vi "DMSV.main.vi"() -> ()   [LabVIEW 2014, in "DMSViewer.lvlib"]
doc: "Displays node and processs information as well as status of CS systems.\n\nHistory: 16-FEB-2006, Dietrich Beck\n\nCopyright (C)\nGesellschaft für Schwerionenforschung, GSI\nPlanckstr. 1\n64291 Darmstadt\nGermany\n\nContact: D.Beck@gsi.de \n\nThis program is free software; you can redistribute it and/or modify it under the terms of the \nGNU General Public License as published by the Free Software Foundation; either version 2 of the license, or (at your option) any later version.\n\nThis program is distributed in the hope that it will be useful, but WITHOUT ANY WARRANTY; without even the implied warranty of MERCHANTABILITY or FITNESS FOR A PARTICULAR PURPOSE. See the GNU General License for more details (http://www.gnu.org).\n\nGesellschaft für Schwerionenforschung, GSI\nPlanckstr. 1, 64291 Darmstadt, Germany\nFor all questions and ideas contact D. Beck.\nLast update: 16-DEC-2005"
uses:
  DMSViewer.lvlib
  CSlibraries-extern/DimLVEvent/LVDimInterface/LVDimInterface.dim service type.ctl
  CSlibraries/UtilityLib/UtilityLib.valueStatus.ctl
  CSlibraries-extern/DimLVEvent/LVDimInterface/LVDimInterface.dic_info_service_notifier.vi
  CSlibraries-extern/DimLVEvent/LVDimInterface/LVDimInterface.lvlib
  CSlibraries/UtilityLib/UtilityLib.lvlib
panel:
  out "nameAndVersion":string
  out "domainMessage":string
  in  "ShowCSSystems":bool
  out "CSSystems":i32(listbox)=-1
  out "noLink":bool
  in  "DomainName":string="KSTest"
  in  "setDomain":bool
  in  "Nodes":i32(listbox)
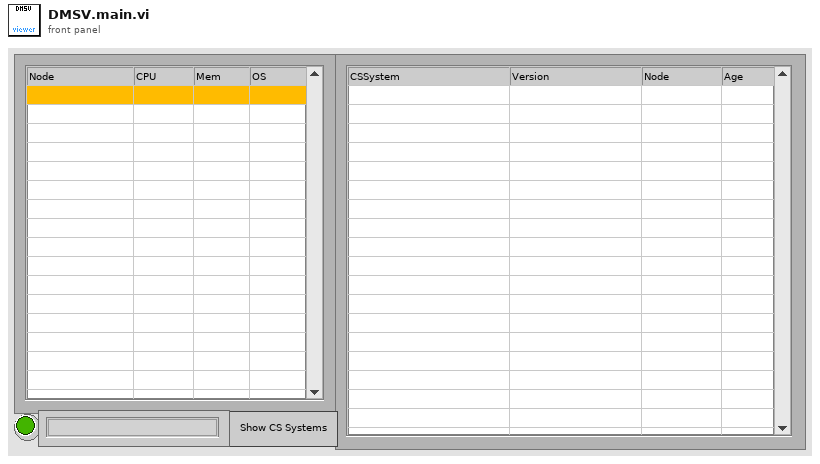
[diagram p1: front panel]
types:
  T1 = typedef "UtilityLib.lvlib/UtilityLib.valueStatus.ctl" = enum16{"no info available", "stand by/off", "on", "warning", "alarm/malfunction", "not implemented", "user action required", "important information", "system default", "control default", "indicator default", "button default"}
  T2 = enum32{"invalid app kind", "Development System", "Run Time System", "Student Edition", "Embedded LabVIEW", "Evaluation", "Custom"}
  T3 = typedef "LVDimInterface.lvlib/LVDimInterface.dim service type.ctl" = u16
  T4 = typedef "LVRectTypeDef.ctl" = cluster{"Left":i16, "Top":i16, "Right":i16, "Bottom":i16}
  T5 = typedef "LVPointTypeDef.ctl" = cluster{"Horizontal":i16, "Vertical":i16}
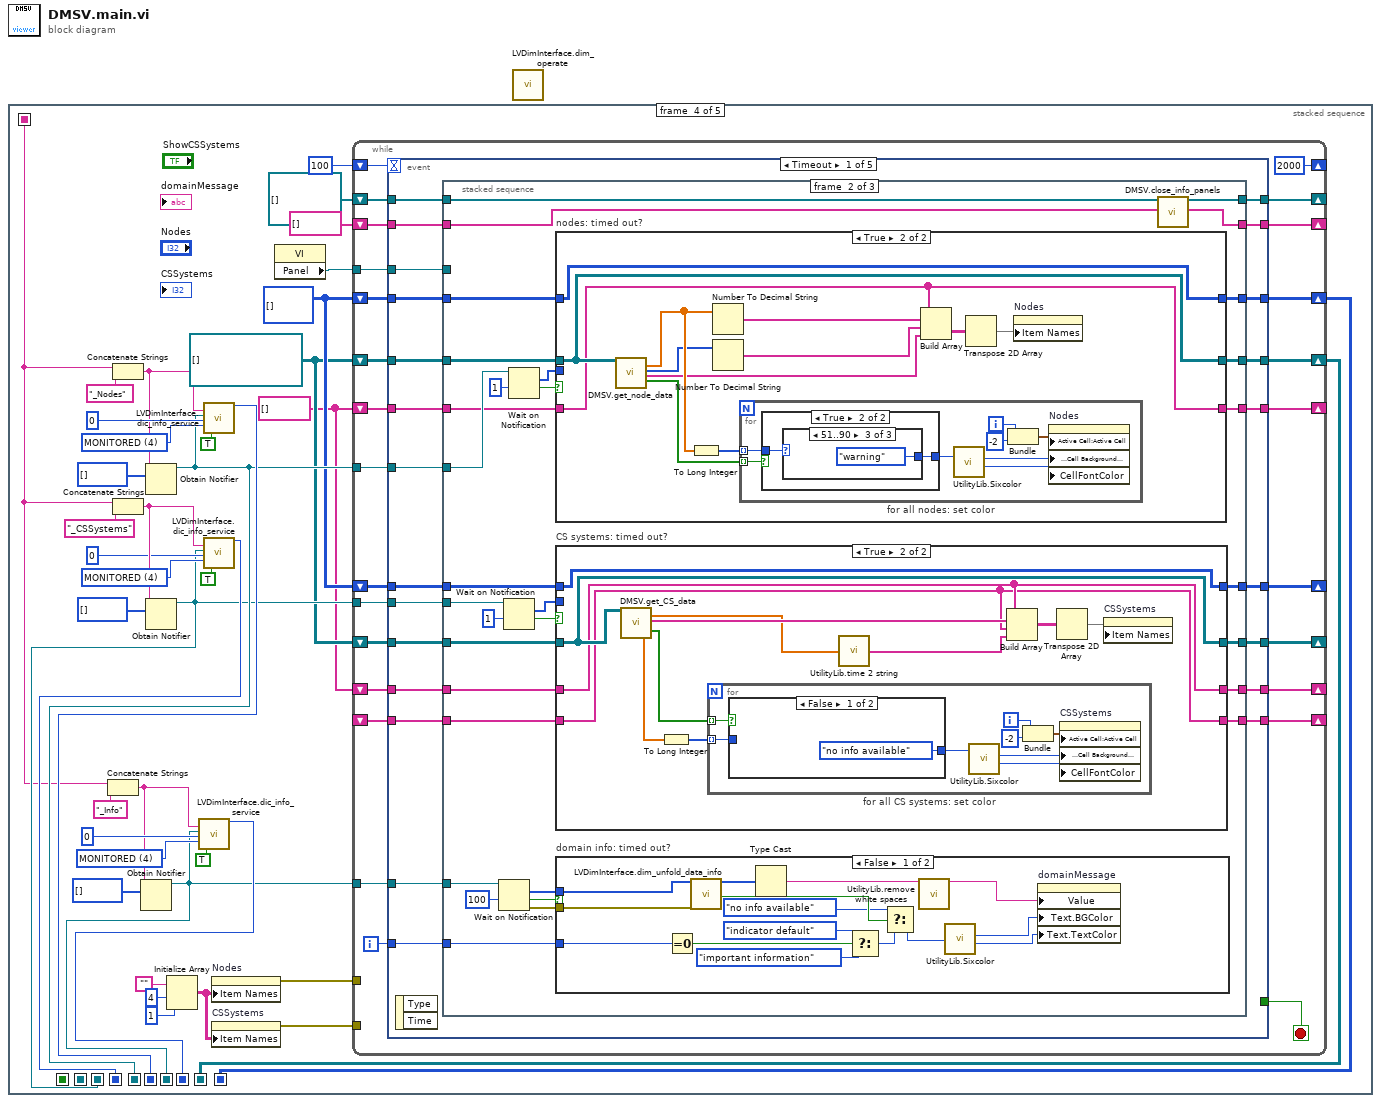
[diagram p0: block diagram]
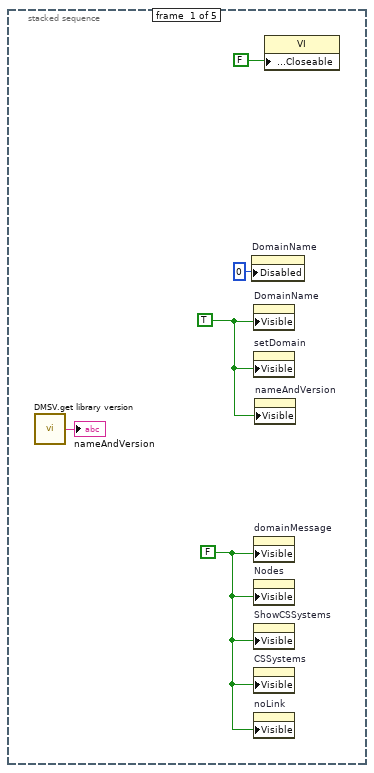
[diagram p2: hidden frame]
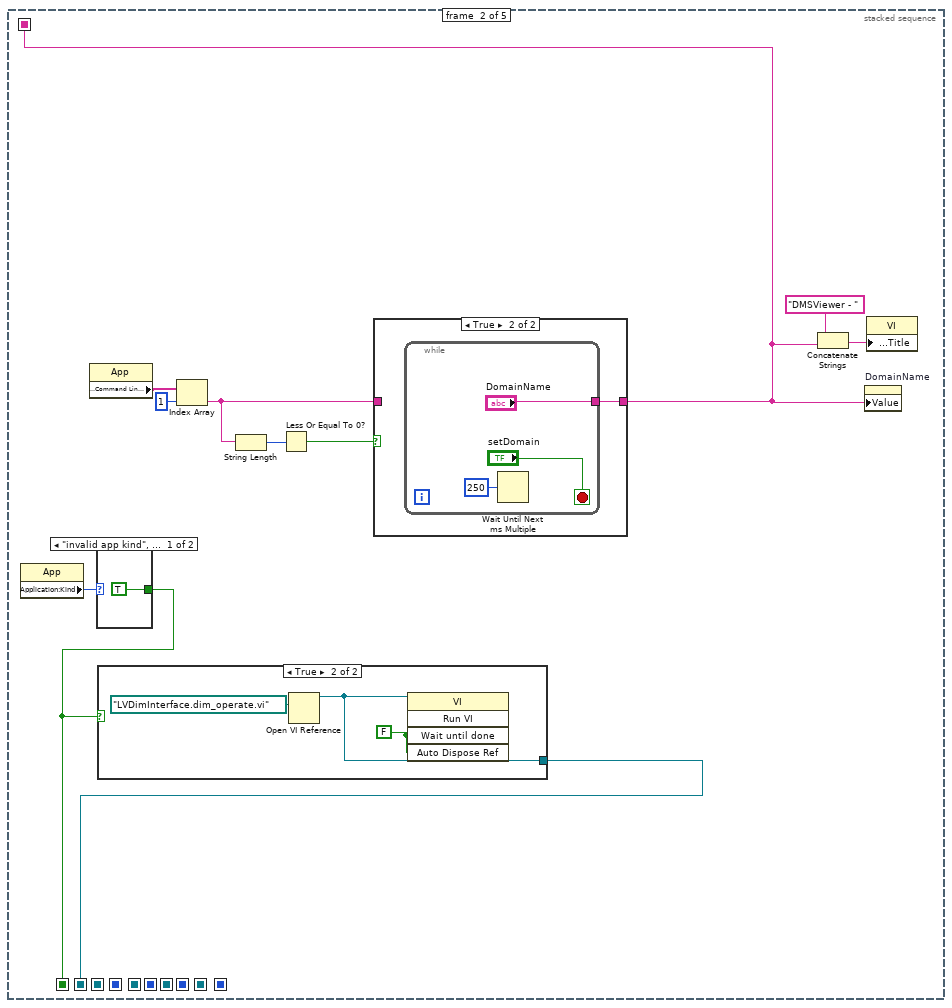
[diagram p3: hidden frame]
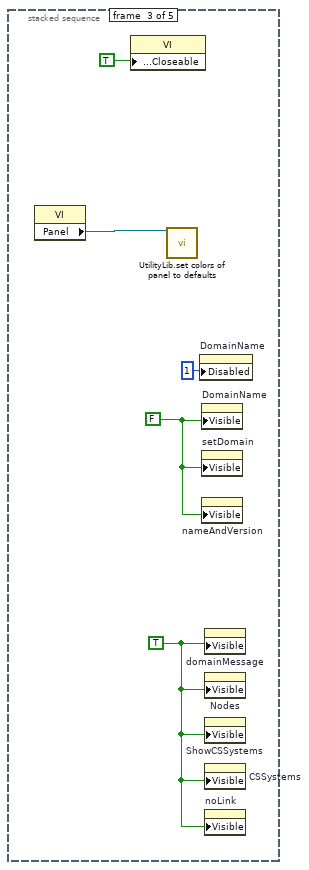
[diagram p7: hidden frame]
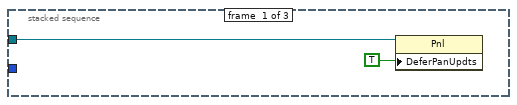
[diagram p8: hidden frame]
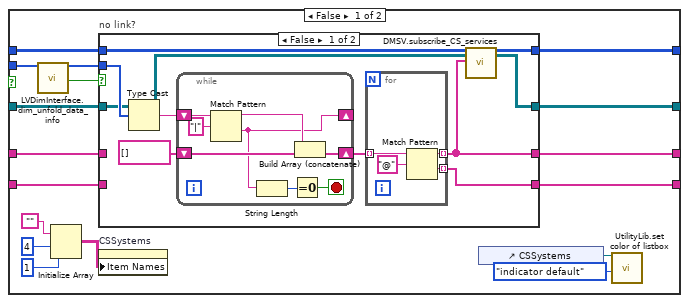
[diagram p10: hidden frame]
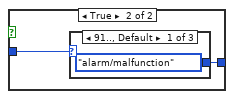
[diagram p12: hidden frame]
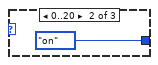
[diagram p13: hidden frame]
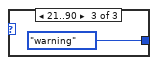
[diagram p14: hidden frame]
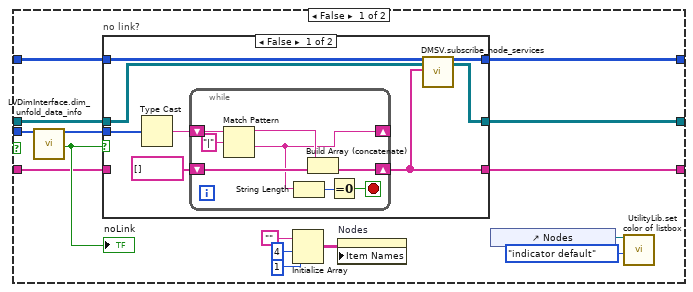
[diagram p15: hidden frame]
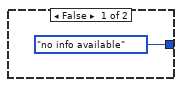
[diagram p17: hidden frame]
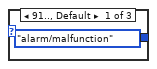
[diagram p18: hidden frame]
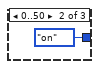
[diagram p19: hidden frame]
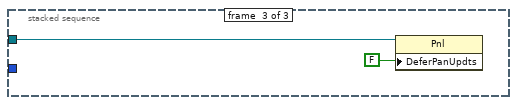
[diagram p20: hidden frame]
diagram:
  n1 = stacked-sequence {
    seq-local: [_ w7 _ _ _] -> [_ _ _ w33 _]
    seq-local: [_ w9 _ _ _] -> [_ _ _ _ w398]
    seq-local: [_ w11 _ _ _] -> [_ _ _ _ w397]
    seq-local: [_ _ _ w54 _] -> [_ _ _ _ w394]
    seq-local: [_ _ _ w59 _] -> [_ _ _ _ w396]
    seq-local: [_ _ _ w56 _] -> [_ _ _ _ w392]
    seq-local: [_ _ _ w55 _] -> [_ _ _ _ w393]
    seq-local: [_ _ _ w47 _] -> [_ _ _ _ w389]
    seq-local: [_ _ _ w46 _] -> [_ _ _ _ w390]
    seq-local: [_ _ _ w31 _] -> [_ _ _ _ w387]
    seq-local: [_ _ _ w32 _] -> [_ _ _ _ w386]
    frame #0 {
      w4 = FALSE ("Visible")
      w1 = TRUE ("Visible")
      n2 = call "DMSV.get library version.vi"() -> ("nameAndVersion"=→"nameAndVersion":string)  [unwired: 1 in]
      n3 = property on="DomainName" class="Str"("Disabled"=u8 0) -> ()  [unwired: 2 in, 2 out]
      n4 = property on="DomainName" class="Str"("Visible"=w1) -> ()  [unwired: 2 in, 2 out]
      n5 = property on="setDomain" class="Bool"("Visible"=w1) -> ()  [unwired: 2 in, 2 out]
      n6 = property on="domainMessage" class="Str"("Visible"=w4) -> ()  [unwired: 2 in, 2 out]
      n7 = property on="Nodes" class="MCListbox (strict)"("Visible"=w4) -> ()  [unwired: 2 in, 2 out]
      n8 = property on="ShowCSSystems" class="Bool (strict)"("Visible"=w4) -> ()  [unwired: 2 in, 2 out]
      n9 = property on="CSSystems" class="MCListbox (strict)"("Visible"=w4) -> ()  [unwired: 2 in, 2 out]
      n10 = property on="noLink" class="Bool (strict)"("Visible"=w4) -> ()  [unwired: 2 in, 2 out]
      n11 = property on="nameAndVersion" class="Str"("Visible"=w1) -> ()  [unwired: 2 in, 2 out]
      n12 = property class="VI"("Front Panel.Closeable"=FALSE ("Front Panel Window:Closeable")) -> ()  [unwired: 2 in, 2 out]
    }
    frame #1 {
      n13 = property on="Property Node" class="App"() -> ("Application:Kind"=w10:T2)  [unwired: 2 in, 2 out]
      n14 = property on="Property Node" class="App"() -> ("Application:Command Line Arguments"=w16:string[])  [unwired: 2 in, 2 out]
      n15 = case shown="\"invalid app kind\", Default" w10 {
        tunnel: [TRUE _] -> w9
        frame "invalid app kind", Default {
        }
        frame "Development System" {
        }
      }
      n16 = case shown="True" w9 {
        tunnel: [_ w18] -> w11
        frame False {
        }
        frame True {
          w19 = FALSE ("Wait until done")
          n17 = Open VI Reference(vi path=path "LVDimInterface.dim_operate.vi") -> (vi reference=w18:refnum<vi>)  [unwired: 5 in, 1 out]
          n18 = invoke on="Invoke Node" class="VI" method="Run VI"(reference=w18, "Wait until done"=w19, "Auto Dispose Ref"=w19) -> ()  [unwired: 2 in, 5 out]
        }
      }
      n19 = Index Array(array=w16, index=1) -> (element=w12:string)
      n20 = String Length(string=w12) -> (length=w14:i32)
      n21 = Less Or Equal To 0?(x=w14) -> (x <= 0?=w13:bool)
      n22 = case shown="True" w13 {
        tunnel: [w21 w22] -> w7
        tunnel: w12 -> [w21 _]
        frame False {
        }
        frame True {
          n23 = while {
            tunnel: ["DomainName"] -> w22
            stop <- "setDomain" stop-if-true
            n24 = Wait Until Next ms Multiple(millisecond multiple=u32 250) -> ()  [unwired: 1 out]
          }
        }
      }
      n25 = Concatenate Strings("DMSViewer - " ("string"), w7) -> (w8:string)
      n26 = property on="DomainName" class="Str"("Value"=w7) -> ()  [unwired: 2 in, 2 out]
      n27 = property on="Property Node" class="VI"("Front Panel Window:Title"=w8) -> ()  [unwired: 2 in, 2 out]
    }
    frame #2 {
      w29 = TRUE ("Visible")
      w26 = FALSE ("Visible")
      n28 = property on="Property Node" class="VI"() -> ("Panel"=w28:refnum<vi>)  [unwired: 2 in, 2 out]
      n29 = property class="VI"("Front Panel.Closeable"=TRUE ("Front Panel Window:Closeable")) -> ()  [unwired: 2 in, 2 out]
      n30 = call "UtilityLib.set colors of panel to defaults.vi"("Front Panel"=w28) -> ()  [unwired: 18 in, 1 out]
      n31 = property on="DomainName" class="Str"("Disabled"=u8 1) -> ()  [unwired: 2 in, 2 out]
      n32 = property on="DomainName" class="Str"("Visible"=w26) -> ()  [unwired: 2 in, 2 out]
      n33 = property on="setDomain" class="Bool"("Visible"=w26) -> ()  [unwired: 2 in, 2 out]
      n34 = property on="nameAndVersion" class="Str"("Visible"=w26) -> ()  [unwired: 2 in, 2 out]
      n35 = property on="domainMessage" class="Str"("Visible"=w29) -> ()  [unwired: 2 in, 2 out]
      n36 = property on="Nodes" class="MCListbox (strict)"("Visible"=w29) -> ()  [unwired: 2 in, 2 out]
      n37 = property on="ShowCSSystems" class="Bool (strict)"("Visible"=w29) -> ()  [unwired: 2 in, 2 out]
      n38 = property on="CSSystems" class="MCListbox (strict)"("Visible"=w29) -> ()  [unwired: 2 in, 2 out]
      n39 = property on="noLink" class="Bool (strict)"("Visible"=w29) -> ()  [unwired: 2 in, 2 out]
    }
    frame #3 {
      w36 = T3 4 items=["ONCE_ONLY"=1, "TIMED"=2, "MONITORED"=4] ("serviceType")
      w43 = string[] []
      w51 = T3 4 items=["ONCE_ONLY"=1, "TIMED"=2, "MONITORED"=4] ("serviceType")
      w44 = refnum<notifier>[][] [] ("nodeNotifiers (out)")
      w45 = i32[][] [] ("nodeServices (out)")
      w60 = T3 4 items=["ONCE_ONLY"=1, "TIMED"=2, "MONITORED"=4] ("serviceType")
      n40 = Concatenate Strings(w33, "_Info" ("string")) -> (w34:string)
      n41 = Concatenate Strings(w33, "_Nodes" ("string")) -> (w57:string)
      n42 = Concatenate Strings(w33, "_CSSystems" ("string")) -> (w53:string)
      n43 = Obtain Notifier(name (unnamed)=w34, notification data type=i8[] []) -> (notifier out=w31:refnum<notifier>)  [unwired: 2 in, 2 out]
      n44 = Obtain Notifier(name (unnamed)=w57, notification data type=i8[] []) -> (notifier out=w54:refnum<notifier>)  [unwired: 2 in, 2 out]
      n45 = Obtain Notifier(name (unnamed)=w53, notification data type=i8[] []) -> (notifier out=w46:refnum<notifier>)  [unwired: 2 in, 2 out]
      n46 = Initialize Array("" ("Empty String Constant"), 4 ("dimension size"), 1 ("dimension size")) -> (w42:string[][])
      n47 = call-poly "LVDimInterface.dic_info_service.vi"("serviceName"=w34, "notifierRef"=w31, "timeout [s]"=0, "serviceType"=w36, "stamped"=TRUE) -> ("callBackID"=w32:i32)  [unwired: 13 in, 1 out]
      n48 = call-poly "LVDimInterface.dic_info_service.vi"("serviceName"=w57, "notifierRef"=w54, "timeout [s]"=0, "serviceType"=w60, "stamped"=TRUE) -> ("callBackID"=w59:i32)  [unwired: 13 in, 1 out]
      n49 = call-poly "LVDimInterface.dic_info_service.vi"("serviceName"=w53, "notifierRef"=w46, "timeout [s]"=0, "serviceType"=w51, "stamped"=TRUE) -> ("callBackID"=w47:i32)  [unwired: 13 in, 1 out]
      n50 = property on="Nodes" class="MCListbox (strict)"("Item Names"=w42) -> (error out=w69:errorcluster)  [unwired: 2 in, 1 out]
      n51 = property on="CSSystems" class="MCListbox (strict)"("Item Names"=w42) -> (error out=w41:errorcluster)  [unwired: 2 in, 1 out]
      n52 = property on="Property Node" class="VI"() -> ("Panel"=w40:refnum<vi>)  [unwired: 2 in, 2 out]
      n53 = while {
        shift-right: [w94] -> _
        shift-left: refnum<vi>[] [] -> [w95]
        tunnel: w69 -> [_]
        shift-right: [2000] -> _
        shift-left: 100 -> [w92]
        shift-right: [w90] -> _
        shift-left: string[] [] -> [w91]
        tunnel: w54 -> [w89]
        shift-right: [w88] -> w55
        shift-left: w45 -> [w86]
        shift-right: [w87] -> w56
        shift-left: w44 -> [w85]
        shift-right: [w84] -> _
        shift-left: w43 -> [w83]
        tunnel: w46 -> [w82]
        shift-right: [w80] -> _
        shift-left: w45 -> [w77]
        shift-right: [w79] -> _
        shift-left: w44 -> [w78]
        shift-right: [w81] -> _
        shift-left: w43 -> [w71]
        tunnel: w41 -> [_]
        shift-right: [w76] -> _
        shift-left: _ -> [w75]
        tunnel: w40 -> [w74]
        tunnel: w31 -> [w73]
        i -> [w72]
        stop <- w96 stop-if-true
        n54 = event shown="[0] Timeout" {
          selector: _ -> [_ _ _ _ _]
          dyn-events: _ -> [_ _ _ _ _]
          timeout: w92 -> [_ _ _ _ _]
          tunnel: [_ _ _ _ TRUE ("EXIT")] -> w96
          tunnel: w95 -> [w118 w310 w323 w365 w383]
          tunnel: [w119 w310 w322 w365 refnum<vi>[] []] -> w94
          tunnel: w91 -> [w117 w309 w318 w364 w381]
          tunnel: [w116 w309 w319 w364 w381] -> w90
          tunnel: w89 -> [w115 _ _ _ _]
          tunnel: [w114 w308 w314 w363 w380] -> w88
          tunnel: [w113 w307 w313 w362 w379] -> w87
          tunnel: w86 -> [w112 w308 w314 w363 w380]
          tunnel: w85 -> [w111 w307 w313 w362 w379]
          tunnel: [w110 w306 w312 w358 w378] -> w84
          tunnel: w83 -> [w109 w306 w312 w358 w378]
          tunnel: w82 -> [w108 _ _ _ _]
          tunnel: [w103 w303 w317 w359 w377] -> w81
          tunnel: [w107 w305 w316 w361 w376] -> w80
          tunnel: [w105 w304 w315 w360 w375] -> w79
          tunnel: w78 -> [w104 w304 w315 w360 w375]
          tunnel: w77 -> [w106 w305 w316 w361 w376]
          tunnel: [w101 w302 w311 w356 w374] -> w76
          tunnel: w75 -> [w100 w302 w311 w356 w374]
          tunnel: w74 -> [w99 _ _ _ _]
          tunnel: w73 -> [w98 _ _ _ _]
          tunnel: w72 -> [w97 _ _ _ _]
          tunnel: w71 -> [w102 w303 w317 w359 w377]
          event Timeout {
            n55 = event-data() -> ()  [unwired: 1 in, 2 out]
            n56 = stacked-sequence {
              tunnel: [_ w153 _] -> w119
              tunnel: w118 -> [_ w152 _]
              tunnel: w117 -> [_ w151 _]
              tunnel: [_ w150 _] -> w116
              tunnel: w115 -> [_ w149 _]
              tunnel: [_ w145 _] -> w114
              tunnel: [_ w144 _] -> w113
              tunnel: w112 -> [_ w143 _]
              tunnel: w111 -> [_ w142 _]
              tunnel: [_ w141 _] -> w110
              tunnel: w109 -> [_ w140 _]
              tunnel: w108 -> [_ w139 _]
              tunnel: [_ w137 _] -> w107
              tunnel: w106 -> [_ w136 _]
              tunnel: [_ w135 _] -> w105
              tunnel: w104 -> [_ w134 _]
              tunnel: [_ w133 _] -> w103
              tunnel: w102 -> [_ w132 _]
              tunnel: [_ w129 _] -> w101
              tunnel: w100 -> [_ w128 _]
              tunnel: w99 -> [w120 _ w298]
              tunnel: w98 -> [_ w127 _]
              tunnel: w97 -> [_ w122 _]
              frame #0 {
                n57 = property on="Property Node" class="Pnl"(reference=w120, "DeferPanUpdts"=TRUE ("Defer Panel Updates")) -> ()  [unwired: 1 in, 2 out]
              }
              frame #1 {
                n58 = Wait on Notification(notifier=w127, timeout in ms (-1)=100) -> (notification=w126:i8[], timed out?=w123:bool, error out=w125:errorcluster)  [unwired: 2 in, 1 out]
                n59 = Wait on Notification(notifier=w139, timeout in ms (-1)=1) -> (notification=w131:i8[], timed out?=w130:bool)  [unwired: 2 in, 2 out]
                n60 = Wait on Notification(notifier=w149, timeout in ms (-1)=1) -> (notification=w146:i8[], timed out?=w147:bool)  [unwired: 2 in, 2 out]
                n61 = case "nodes: timed out?" shown="True" w147 {
                  tunnel: w146 -> [w252 _]
                  tunnel: [w249 w274] -> w145
                  tunnel: [w248 w280] -> w144
                  tunnel: w143 -> [w247 w274]
                  tunnel: w142 -> [w246 w280]
                  tunnel: [w245 w273] -> w141
                  tunnel: w140 -> [w244 w273]
                  frame False {
                    n62 = call "LVDimInterface.dim_unfold_data_info.vi"("rawData"=w252) -> ("data"=w251:i8[], "no link"=w250:bool)  [unwired: 8 in, 9 out]
                    "noLink" <- w250
                    n63 = case "no link?" shown="False" w250 {
                      tunnel: w251 -> [w260 _]
                      tunnel: [w257 w271] -> w249
                      tunnel: [w256 w270] -> w248
                      tunnel: w247 -> [w255 w271]
                      tunnel: w246 -> [w254 w270]
                      tunnel: [w253 w269] -> w245
                      tunnel: w244 -> [_ w269]
                      frame False {
                        n64 = Type Cast(x=w260) -> (*(type *) &x=w259:string)  [unwired: 1 in]
                        n65 = while {
                          shift-right: [w263] -> w253
                          shift-left: string[] [] -> [w264]
                          shift-right: [w261] -> _
                          shift-left: w259 -> [w268]
                          stop <- w266 stop-if-true
                          n66 = Match Pattern(string=w268, regular expression="|") -> (before substring=w262:string, after substring=w261:string)  [unwired: 1 in, 2 out]
                          n67 = String Length(string=w261) -> (length=w267:i32)
                          n68 = Build Array (concatenate)(w262, w264) -> (w263:string[])
                          n69 = Equal To 0?(x=w267) -> (x = 0?=w266:bool)
                        }
                        n70 = call "DMSV.subscribe_node_services.vi"("nodeServices"=w255, "nodeNotifiers"=w254, "nodes"=w253) -> ("nodeServices (out)"=w257:i32[][], "nodeNotifiers (out)"=w256:refnum<notifier>[][])  [unwired: 14 in, 1 out]
                      }
                      frame True {
                      }
                    }
                    n71 = Initialize Array("" ("Empty String Constant"), 4 ("dimension size"), 1 ("dimension size")) -> (w240:string[][])
                    n72 = property on="Nodes" class="MCListbox (strict)"("Item Names"=w240) -> ()  [unwired: 2 in, 2 out]
                    n73 = control-ref of="Nodes"() -> (w238:refnum<vi>)
                    n74 = call "UtilityLib.set color of listbox.vi"("listboxRef"=w238, "valueStatus"=UtilityLib.valueStatus."indicator default" ("isControl?")) -> ()  [unwired: 17 in, 1 out]
                  }
                  frame True {
                    n75 = call "DMSV.get_node_data.vi"("nodeNotifiers"=w280) -> ("CPU"=w283:sgl[], "Mem"=w282:i32[], "OS"=w281:string[], "link?"=w272:bool[])  [unwired: 13 in, 2 out]
                    n76 = To Long Integer(number=w283) -> (32bit integer=w276:i32[])
                    n77 = Number To Decimal String(number=w283) -> (decimal integer string=w279:string[])  [unwired: 1 in]
                    n78 = Number To Decimal String(number=w282) -> (decimal integer string=w278:string[])  [unwired: 1 in]
                    n79 = for "for all nodes: set color" {
                      tunnel: w276 -> [w291] mode=indexing
                      tunnel: w272 -> [w290] mode=indexing
                      i -> [w284]
                      n80 = case shown="True" w290 {
                        tunnel: w291 -> [_ w294]
                        tunnel: [UtilityLib.valueStatus."no info available" ("valueStatus") w293] -> w285
                        frame False {
                        }
                        frame True {
                          n81 = case shown="51..90" w294 {
                            tunnel: [UtilityLib.valueStatus."alarm/malfunction" ("valueStatus") UtilityLib.valueStatus."on" ("valueStatus") UtilityLib.valueStatus."warning" ("valueStatus")] -> w293
                            frame 91.., Default {
                            }
                            frame 0..50 {
                            }
                            frame 51..90 {
                            }
                          }
                        }
                      }
                      n82 = call "UtilityLib.Sixcolor.vi"("State"=w285) -> ("elementBackground"=w287:u32, "elementText"=w286:u32)  [unwired: 2 in, 2 out]
                      n83 = Bundle(w284, -2) -> (w289:cluster{i32, i32})  [unwired: 1 in]
                      n84 = property on="Nodes" class="MCListbox (strict)"("Active Cell:Active Cell"=w289, "Active Cell:Cell Background Color"=w287, "CellFontColor"=w286) -> ()  [unwired: 2 in, 2 out]
                    }
                    n85 = Build Array(w273, w279, w278, w281) -> (w275:string[][])
                    n86 = Transpose 2D Array(2D array=w275) -> (transposed array=w277:string[][])
                    n87 = property on="Nodes" class="MCListbox (strict)"("Item Names"=w277) -> ()  [unwired: 2 in, 2 out]
                  }
                }
                n88 = case "CS systems: timed out?" shown="True" w130 {
                  tunnel: [w183 w219] -> w137
                  tunnel: w136 -> [w184 w219]
                  tunnel: [w179 w218] -> w135
                  tunnel: w134 -> [w180 w218]
                  tunnel: [w177 w217] -> w133
                  tunnel: w132 -> [w178 w217]
                  tunnel: w131 -> [w182 _]
                  tunnel: [w172 w215] -> w129
                  tunnel: w128 -> [w171 w215]
                  frame False {
                    n89 = call "LVDimInterface.dim_unfold_data_info.vi"("rawData"=w182) -> ("data"=w185:i8[], "no link"=w181:bool)  [unwired: 8 in, 9 out]
                    n90 = Initialize Array("" ("Empty String Constant"), 4 ("dimension size"), 1 ("dimension size")) -> (w176:string[][])
                    n91 = case "no link?" shown="False" w181 {
                      tunnel: w185 -> [w193 _]
                      tunnel: w184 -> [w192 w211]
                      tunnel: [w191 w211] -> w183
                      tunnel: w180 -> [w190 w210]
                      tunnel: [w189 w210] -> w179
                      tunnel: [w187 w209] -> w177
                      tunnel: w178 -> [_ w209]
                      tunnel: [w186 w208] -> w172
                      tunnel: w171 -> [_ w208]
                      frame False {
                        n92 = Type Cast(x=w193) -> (*(type *) &x=w194:string)  [unwired: 1 in]
                        n93 = while {
                          shift-right: [w202] -> w188
                          shift-left: string[] [] -> [w203]
                          shift-right: [w200] -> _
                          shift-left: w194 -> [w207]
                          stop <- w205 stop-if-true
                          n94 = Match Pattern(string=w207, regular expression="|") -> (before substring=w201:string, after substring=w200:string)  [unwired: 1 in, 2 out]
                          n95 = String Length(string=w200) -> (length=w206:i32)
                          n96 = Equal To 0?(x=w206) -> (x = 0?=w205:bool)
                          n97 = Build Array (concatenate)(w201, w203) -> (w202:string[])
                        }
                        n98 = for {
                          tunnel: w188 -> [w199] mode=indexing
                          tunnel: [w197] -> w187 mode=indexing
                          tunnel: [w196] -> w186 mode=indexing
                          n99 = Match Pattern(string=w199, regular expression="@") -> (before substring=w197:string, after substring=w196:string)  [unwired: 1 in, 2 out]
                        }
                        n100 = call "DMSV.subscribe_CS_services.vi"("csServices"=w192, "csNotifiers"=w190, "csSystems"=w187) -> ("csServices (out)"=w191:i32[][], "csNotifiers (out)"=w189:refnum<notifier>[][])  [unwired: 14 in, 1 out]
                      }
                      frame True {
                      }
                    }
                    n101 = property on="CSSystems" class="MCListbox (strict)"("Item Names"=w176) -> ()  [unwired: 2 in, 2 out]
                    n102 = control-ref of="CSSystems"() -> (w170:refnum<vi>)
                    n103 = call "UtilityLib.set color of listbox.vi"("listboxRef"=w170, "valueStatus"=UtilityLib.valueStatus."indicator default" ("isControl?")) -> ()  [unwired: 17 in, 1 out]
                  }
                  frame True {
                    n104 = call "DMSV.get_CS_data.vi"("csNotifiers"=w218) -> ("lastUpdated"=w216:dbl[], "age"=w214:dbl[], "version"=w223:string[], "link?"=w213:bool[])  [unwired: 13 in, 2 out]
                    n105 = To Long Integer(number=w216) -> (32bit integer=w212:i32[])
                    n106 = for "for all CS systems: set color" {
                      tunnel: w212 -> [w225] mode=indexing
                      tunnel: w213 -> [w226] mode=indexing
                      i -> [w227]
                      n107 = case shown="False" w226 {
                        tunnel: w225 -> [_ w234]
                        tunnel: [UtilityLib.valueStatus."no info available" ("valueStatus") w233] -> w224
                        frame False {
                        }
                        frame True {
                          n108 = case shown="91.., Default" w234 {
                            tunnel: [UtilityLib.valueStatus."alarm/malfunction" ("valueStatus") UtilityLib.valueStatus."on" ("valueStatus") UtilityLib.valueStatus."warning" ("valueStatus")] -> w233
                            frame 91.., Default {
                            }
                            frame 0..20 {
                            }
                            frame 21..90 {
                            }
                          }
                        }
                      }
                      n109 = call "UtilityLib.Sixcolor.vi"("State"=w224) -> ("elementBackground"=w230:u32, "elementText"=w231:u32)  [unwired: 2 in, 2 out]
                      n110 = Bundle(w227, -2) -> (w228:cluster{i32, i32})  [unwired: 1 in]
                      n111 = property on="CSSystems" class="MCListbox (strict)"("Active Cell:Active Cell"=w228, "Active Cell:Cell Background Color"=w230, "CellFontColor"=w231) -> ()  [unwired: 2 in, 2 out]
                    }
                    n112 = call "UtilityLib.time 2 string.vi"("time"=w214) -> ("timeString"=w222:string[])
                    n113 = Build Array(w217, w223, w215, w222) -> (w221:string[][])
                    n114 = Transpose 2D Array(2D array=w221) -> (transposed array=w220:string[][])
                    n115 = property on="CSSystems" class="MCListbox (strict)"("Item Names"=w220) -> ()  [unwired: 2 in, 2 out]
                  }
                }
                n116 = case "domain info: timed out?" shown="False" w123 {
                  tunnel: w126 -> [w168 _]
                  tunnel: w125 -> [w167 _]
                  tunnel: w122 -> [w162 _]
                  frame False {
                    n117 = Equal To 0?(x=w162) -> (x = 0?=w164:bool)
                    n118 = call "LVDimInterface.dim_unfold_data_info.vi"("rawData"=w168, "error in (no error)"=w167) -> ("data"=w166:i8[], "no link"=w157:bool)  [unwired: 7 in, 9 out]
                    n119 = Type Cast(x=w166) -> (*(type *) &x=w165:string)  [unwired: 1 in]
                    n120 = Select(t=UtilityLib.valueStatus."indicator default" ("State"), s=w164, f=UtilityLib.valueStatus."important information" ("State")) -> (s? t:f=w156:T1)
                    n121 = Select(t=UtilityLib.valueStatus."no info available" ("State"), s=w157, f=w156) -> (s? t:f=w155:T1)
                    n122 = call "UtilityLib.remove white spaces.vi"("string with blanks"=w165) -> ("string without white spaces"=w163:string)  [unwired: 14 in, 4 out]
                    n123 = call "UtilityLib.Sixcolor.vi"("State"=w155) -> ("elementBackground"=w159:u32, "elementText"=w158:u32)  [unwired: 2 in, 2 out]
                    n124 = property on="domainMessage" class="Str"("Value"=w163, "Text.BGColor"=w159, "Text.TextColor"=w158) -> ()  [unwired: 2 in, 2 out]
                  }
                  frame True {
                  }
                }
                n125 = call "DMSV.close_info_panels.vi"("infoPanels"=w152, "panel@node"=w151) -> ("infoPanels out"=w153:refnum<vi>[], "panel@node out"=w150:string[])  [unwired: 15 in, 1 out]
              }
              frame #2 {
                n126 = property on="Property Node" class="Pnl"(reference=w298, "DeferPanUpdts"=FALSE ("Defer Panel Updates")) -> ()  [unwired: 1 in, 2 out]
              }
            }
          }
          event "domainMessage": Mouse Down {
            n127 = event-data() -> ()  [unwired: 1 in, 4 out]
            n128 = control-ref of="domainMessage"() -> (w301:refnum<vi>)
            n129 = call "UtilityLib.set color of simple string or numeric.vi"("simpleString"=w301, "valueStatus"=UtilityLib.valueStatus."indicator default" ("isControl?")) -> ()  [unwired: 17 in, 1 out]
          }
          event "Nodes": Double Click {
            n130 = event-data() -> ("Row"=w324:i32)  [unwired: 1 in]
            n131 = Index Array(array=w312, index=w324) -> (element=w320:string)
            n132 = Search 1D Array(1D array=w318, element=w320) -> (index of element=w321:i32)  [unwired: 1 in]
            n133 = case shown="-1" w321 {
              tunnel: w320 -> [_ w335]
              tunnel: w313 -> [_ _]
              tunnel: w324 -> [_ _]
              tunnel: w323 -> [w325 w340]
              tunnel: [w325 w338] -> w322
              tunnel: w318 -> [w326 w337]
              tunnel: [w326 w336] -> w319
              frame 0, Default {
              }
              frame -1 {
                n134 = property on="DomainName" class="Str"() -> ("Value"=w328:string)  [unwired: 2 in, 2 out]
                n135 = Open VI Reference(vi path=path "DMSV.get_pcmon_info.vit", options=0) -> (vi reference=w348:refnum<vi>)  [unwired: 4 in, 1 out]
                n136 = To Variant(anything=w335) -> (Variant=w334:variant)
                n137 = invoke on="Invoke Node" class="VI" method="Ctrl Val.Set"(reference=w348, "Control Name"="node", "Value"=w334) -> (reference out=w333:refnum<vi>, error out=w332:errorcluster)  [unwired: 2 in, 3 out]
                n138 = To Variant(anything=w328) -> (Variant=w327:variant)
                n139 = invoke on="Invoke Node" class="VI" method="Ctrl Val.Set"(reference=w333, error in=w332, "Control Name"="domain", "Value"=w327) -> (reference out=w330:refnum<vi>, error out=w331:errorcluster)  [unwired: 1 in, 3 out]
                n140 = property on="Property Node" class="VI"(reference=w330, error in=w331, "Front Panel Window:Open"=TRUE) -> (reference out=w344:refnum<vi>, error out=w343:errorcluster)
                n141 = invoke on="Invoke Node" class="VI" method="Run VI"(reference=w344, error in=w343, "Wait until done"=FALSE, "Auto Dispose Ref"=FALSE) -> (reference out=w339:refnum<vi>)  [unwired: 1 in, 4 out]
                n142 = Build Array (concatenate)(w337, w335) -> (w336:string[])
                n143 = Build Array (concatenate)(w340, w339) -> (w338:refnum<vi>[])
              }
            }
          }
          event "ShowCSSystems": Value Change {
            w351 = i16 460
            n144 = event-data() -> ()  [unwired: 1 in, 6 out]
            n145 = property on="Property Node" class="VI"() -> ("Front Panel Window:Panel Bounds"=w371:T4)  [unwired: 2 in, 2 out]
            n146 = property on="Property Node" class="VI"() -> ("Front Panel Window:Origin"=w368:T5)  [unwired: 2 in, 2 out]
            n147 = Unbundle By Name(w371) -> ("Right"=w355:i16, "Left"=w354:i16)
            n148 = Subtract(x=w355, y=w354) -> (x-y=w353:i16)
            n149 = Less?(x=w353, y=w351) -> (x < y?=w352:bool)
            n150 = Negate(x=w351) -> (-x=w350:i16)
            n151 = Unbundle By Name(w368) -> ("Horizontal"=w357:i16)
            n152 = Select(t=w351, s=w352, f=w350) -> (s? t:f=w366:i16)
            n153 = Add(x=w355, y=w366) -> (x+y=w370:i16)
            n154 = Bundle By Name(cluster=w368, "Horizontal"=w357) -> (w367:T5)
            n155 = Bundle By Name(cluster=w371, "Right"=w370) -> (w369:T4)
            n156 = property on="Property Node" class="VI"("Front Panel Window:Panel Bounds"=w369) -> ()  [unwired: 2 in, 2 out]
            n157 = property on="Property Node" class="VI"("Front Panel Window:Origin"=w367) -> ()  [unwired: 2 in, 2 out]
          }
          event Panel Close? {
            n158 = event-data() -> ()  [unwired: 1 in, 4 out]
            n159 = for {
              tunnel: w383 -> [w385] mode=indexing
              n160 = invoke on="Invoke Node" class="VI" method="FP.Close"(reference=w385) -> (reference out=w384:refnum<vi>)  [unwired: 2 in, 2 out]
              n161 = Close Reference(reference=w384) -> ()  [unwired: 1 in, 1 out]
            }
            n162 = event-data ("Event Filter Node")("Discard?"=TRUE) -> ()  [unwired: 1 in, 1 out]
          }
        }
      }
    }
    frame #4 {
      n163 = case shown="True" w398 {
        tunnel: w397 -> [_ w406]
        frame False {
        }
        frame True {
          n164 = invoke on="Invoke Node" class="VI" method="Ctrl Val.Set"(reference=w406, "Control Name"="stop", "Value"=TRUE) -> (error out=w408:errorcluster)  [unwired: 2 in, 4 out]
          n165 = flat-sequence {
            tunnel: w406 -> [w411]
            tunnel: w408 -> [w412]
            tunnel: [w412] -> w405
            tunnel: [w411] -> w404
            tunnel: w405 -> [w414]
            tunnel: w404 -> [w413]
            frame #0 {
              n166 = Wait (ms)(milliseconds to wait=u32 1000) -> ()  [unwired: 1 out]
            }
            frame #1 {
              n167 = Close Reference(reference=w413, error in (no error)=w414) -> ()  [unwired: 1 out]
            }
            frame #2 {
              n168 = Quit LabVIEW() -> ()  [unwired: 1 in]
            }
          }
        }
      }
      n169 = call "LVDimInterface.dic_release_service.vi"("callBackID"=w389) -> ("error out"=w391:errorcluster)  [unwired: 18 in]
      n170 = call "LVDimInterface.dic_release_service.vi"("callBackID"=w396) -> ("error out"=w395:errorcluster)  [unwired: 18 in]
      n171 = call "LVDimInterface.dic_release_service.vi"("callBackID"=w386) -> ("error out"=w388:errorcluster)  [unwired: 18 in]
      n172 = Release Notifier(notifier=w390, error in (no error)=w391) -> ()  [unwired: 1 in, 3 out]
      n173 = Release Notifier(notifier=w394, error in (no error)=w395) -> ()  [unwired: 1 in, 3 out]
      n174 = Release Notifier(notifier=w387, error in (no error)=w388) -> ()  [unwired: 1 in, 3 out]
      n175 = for "for all nodes" {
        tunnel: w393 -> [w400] mode=indexing
        tunnel: w392 -> [w399] mode=indexing
        n176 = for "for all services" {
          tunnel: w400 -> [w403] mode=indexing
          tunnel: w399 -> [w402] mode=indexing
          n177 = call "LVDimInterface.dic_release_service.vi"("callBackID"=w403) -> ("error out"=w401:errorcluster)  [unwired: 18 in]
          n178 = Release Notifier(notifier=w402, error in (no error)=w401) -> ()  [unwired: 1 in, 3 out]
        }
      }
    }
  }
  n179 = call "LVDimInterface.dim_operate.vi"() -> ()  [unwired: 20 in]
